vi "Test Load Tree.vi"() -> ()   [LabVIEW 2020, in "CDM-Config.lvlib"]
uses:
  CDM-Config.lvlib
  Config Manager/Config Manager.lvclass/Config Manager.ctl
  Config-JSON/Config-JSON.lvclass
  C:/dev/lv20CE/relink/lv-cdm/CDM-Config/Config Storage/Config Storage.lvclass
  Config Element/Set Owner.vi
  Config Element/Config Element.lvclass
  Config Manager/Config Manager.lvclass
  Config Storage/Config Storage.lvclass
panel:
  in  "Path":path
  in  "Tree":string(tree)
  out "error out":errorcluster
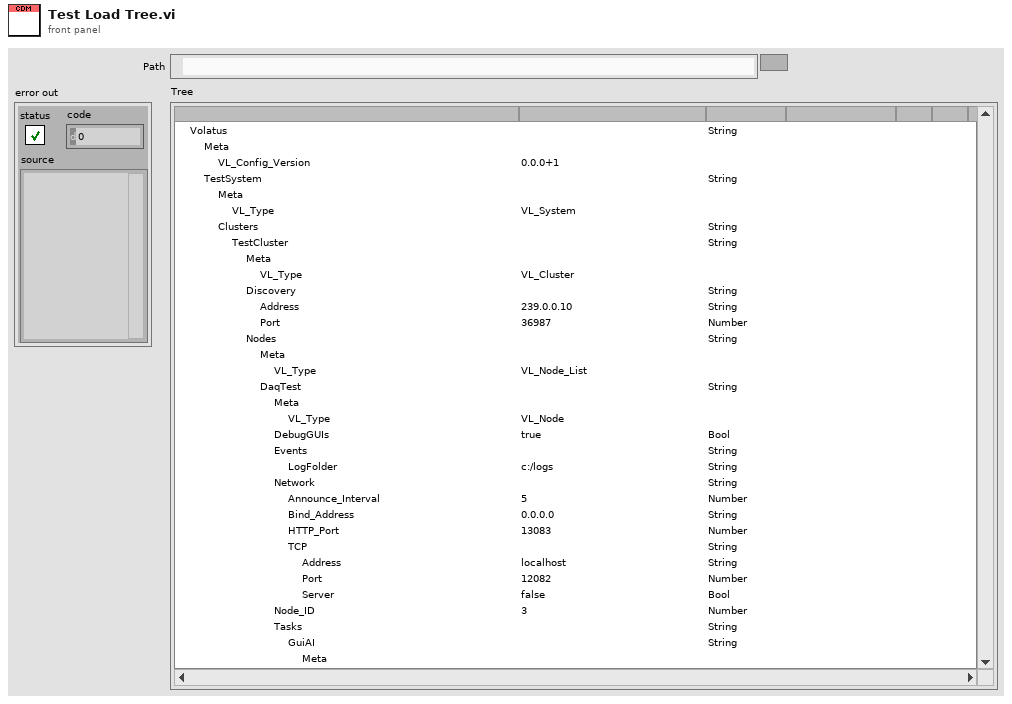
[diagram p1: front panel]
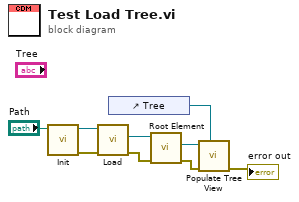
[diagram p0: block diagram]
diagram:
  n1 = call "Init.vi"("Path"="Path") -> ("error out"=w6:errorcluster, "Config-JSON out"=w7:refnum<class "Config-JSON.lvclass">)  [unwired: 9 in]
  n2 = call "Load.vi"("error in (no error)"=w6, "Config Storage in"=w7) -> ("error out"=w5:errorcluster, "Config"=w3:refnum<class "Config Manager.lvclass">)  [unwired: 7 in, 1 out]
  n3 = control-ref of="Tree"() -> (w2:refnum<vi>)
  n4 = call "Root Element.vi"("error in (no error)"=w5, "Config Manager in"=w3) -> ("error out"=w4:errorcluster, "Root Element"=w9:refnum<class "Config Element.lvclass">)  [unwired: 7 in, 1 out]
  n5 = call "Populate Tree View.vi"("Tree"=w2, "error in (no error)"=w4, "Element"=w9) -> ("error out"=→"error out":errorcluster)  [unwired: 8 in]
